vi "Test Base Namer No Extension With Label.vi"(11 "Test Case In":refnum<class "Namer Tests.lvclass">) -> (0 "error out":errorcluster, 3 "Test Case Out":refnum<class "Namer Tests.lvclass">)   [LabVIEW 2020, in "Namer Tests.lvclass"]
uses:
  Namer Tests.lvclass
  C:/Program Files/National Instruments/LabVIEW 2026/vi.lib/Astemes/LUnit/Test Case.lvclass
  Source/Approval Tests/Naming Data/Naming Data.lvclass
  Source/Approval Tests/Namer/Namer.lvclass
  Source/Approval Tests/Naming Data/Naming Data.lvclass/Naming Data.ctl
  <vilib>/Astemes/LUnit/Test Case.lvclass/Test Case.ctl
  4993e8ee-a06a-463a-9684-69129f64d5ce.vi
  15f7ff99-8e41-44be-bd6b-58d836230369.vi
  Source/Approval Tests/Naming Data/Write Test VI Name.vi
  Source/Approval Tests/Naming Data/Write Test Label.vi
  <vilib>/Astemes/LUnit/Core/LUnit Test Case/Private/Append Pass Result.vi
  <vilib>/Astemes/LUnit/Core/LUnit Test Case/Private/Append Fail Result.vi
  4993e8ee-a06a-463a-9684-69129f64d5ce.vi/9c5d11cd-9439-4240-a1ee-d9baace9c924.vi
  15f7ff99-8e41-44be-bd6b-58d836230369.vi/9c5d11cd-9439-4240-a1ee-d9baace9c924.vi
  <vilib>/Astemes/LUnit/Core/LUnit Test Case/Private/Run In UI.vi
  <vilib>/Utility/error.llb/Clear Errors.vi
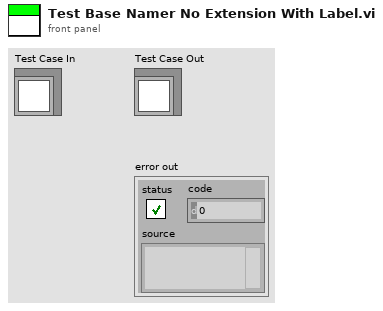
[diagram p1: front panel]
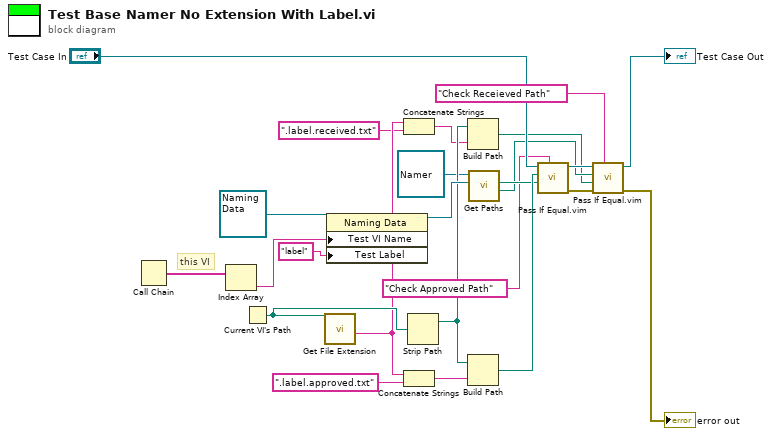
[diagram p0: block diagram]
diagram:
  # "this VI"
  n1 = Call Chain() -> (call chain=w20:string[])
  n2 = Index Array(array=w20) -> (element=w19:string)  [unwired: 1 in]
  n3 = Current VI's Path() -> (path=w17:path)
  n4 = call <vilib>:"Get File Extension.vi"("file"=w17) -> ("filename without extension"=w15:string)  [unwired: 6 in, 4 out]
  n5 = property on="Property Node" class="Naming Data"(reference=refnum<class "Naming Data.lvclass"> refnum ("Naming Data"), "Test VI Name"=w19, "Test Label"="label") -> (reference out=w18:refnum<class "Naming Data.lvclass">)  [unwired: 1 in, 1 out]
  n6 = Concatenate Strings(w15, ".label.received.txt" ("string")) -> (w12:string)
  n7 = Concatenate Strings(w15, ".label.approved.txt" ("string")) -> (w11:string)
  n8 = Strip Path(path=w17) -> (stripped path=w16:path)  [unwired: 1 out]
  n9 = Build Path(base path=w16, name or relative path=w12) -> (appended path=w2:path)
  n10 = Build Path(base path=w16, name or relative path=w11) -> (appended path=w9:path)
  n11 = call-dynamic "Get Paths.vi"("Naming Data"=w18, "Namer in"=refnum<class "Namer.lvclass"> refnum ("Approval Tests:Namer")) -> ("Received Path"=w3:path, "Approved Path"=w8:path)  [unwired: 6 in, 2 out]
  n12 = call "Pass If Equal.vim"("Description"="Check Approved Path" ("Label (VI Title)"), "Actual"=w8, "Expected"=w9, "LUnit Test Case In"="Test Case In") -> ("error out"=w23:errorcluster, "LUnit Test Case Out"=w6:refnum<class "Namer Tests.lvclass">)  [unwired: 6 in]
  n13 = call "Pass If Equal.vim"("Description"="Check Receieved Path" ("Label (VI Title)"), "error in (no error)"=w23, "Actual"=w2, "Expected"=w3, "LUnit Test Case In"=w6) -> ("error out"=→"error out":errorcluster, "LUnit Test Case Out"=→"Test Case Out":refnum<class "Namer Tests.lvclass">)  [unwired: 5 in]
